vi "读取地址和长度.vi"(8 "error in":errorcluster) -> (0 "error out":errorcluster, 1 "return":i32, 2 "data out":u8[](array[numeric]) format="%.0x")   [LabVIEW 2016]
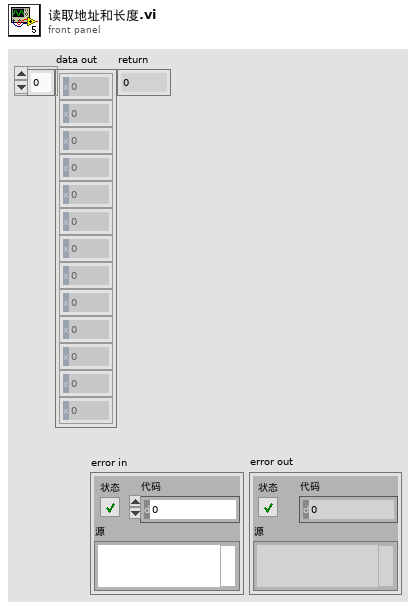
[diagram p1: front panel]
types:
  T1 = cluster{"byCmdType":u8, "bySubCmd":u8, "byPara":u8, "byAddr_h":u8, "byAddr_l":u8, "byAddr_ll":u8, "byLen_h":u8, "byLen_l":u8}
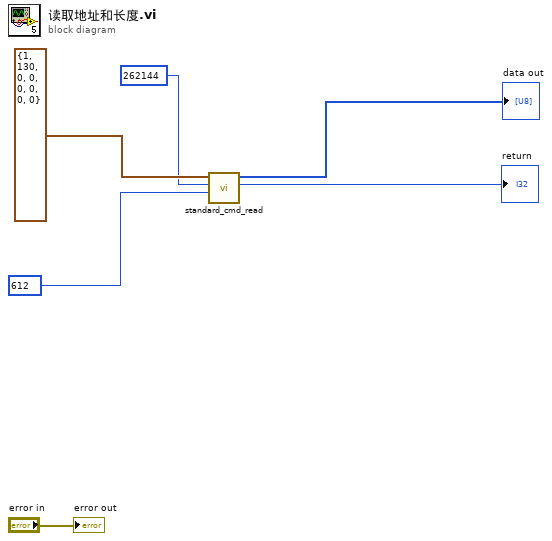
[diagram p0: block diagram]
diagram:
  n1 = call "standard_cmd_read.vi"("dwLen"=u32 612, "dwAddr"=u32 262144, "cmd_std_header_t"=T1 {"byCmdType"=1, "bySubCmd"=130, "byPara"=0, "byAddr_h"=0, "byAddr_l"=0, "byAddr_ll"=0, "byLen_h"=0, "byLen_l"=0}) -> ("return"=→"return":i32, "data out"=→"data out":u8[])  [unwired: 7 in]
  "error out" <- "error in"
